vi "ReadInitParameters.vi"(8 "error in (no error)":errorcluster, 11 "INI Filepath":path) -> (0 "error out":errorcluster, 3 "Init Parameters":T1)   [LabVIEW 2020, in "ClashRoyale.lvclass"]
uses:
  ClashRoyale.lvclass
  InitParameters.ctl
  <vilib>/Utility/config.llb/Read Key (String).vi
  <vilib>/Utility/config.llb/NI_LVConfig.lvlib
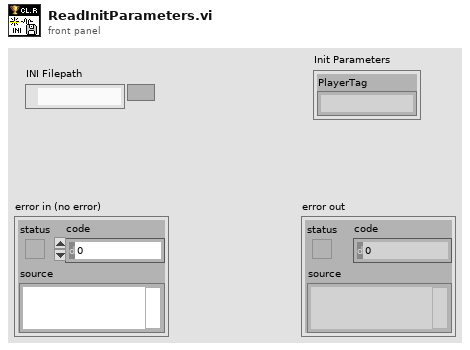
[diagram p1: front panel]
types:
  T1 = typedef "InitParameters.ctl" = cluster{"PlayerTag":string}
  T2 = typedef "NI_LVConfig.lvlib/Config Data RefNum.ctl" = refnum<k1>
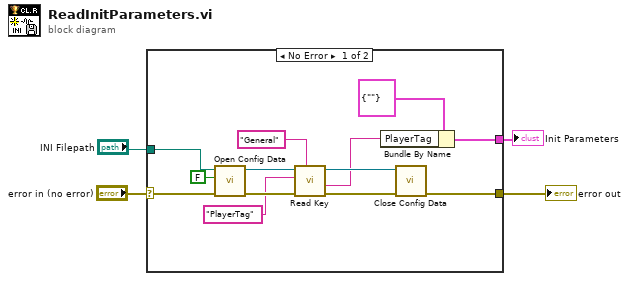
[diagram p0: block diagram]
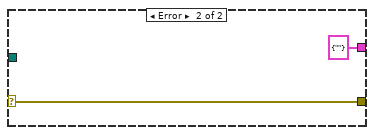
[diagram p2: hidden frame]
diagram:
  n1 = case shown="No Error" "error in (no error)" {
    selector: "error in (no error)" -> [w9 w19]
    tunnel: "INI Filepath" -> [w17 _]
    tunnel: [w8 w19] -> w2
    tunnel: [w5 T1 {"PlayerTag"=""} ("Init Parameters")] -> w1
    frame No Error {
      n2 = call <vilib>:"Open Config Data.vi"("error in (no error)"=w9, "create file if necessary (T)"=FALSE, "configuration file path"=w17) -> ("error out"=w14:errorcluster, "refnum"=w15:T2)  [unwired: 6 in, 1 out]
      n3 = call-poly <vilib>:"Read Key.vi"("section"="General", "error in (no error)"=w14, "key"="PlayerTag", "refnum"=w15) -> ("error out"=w10:errorcluster, "value"=w6:string, "refnum out"=w11:T2)  [unwired: 4 in, 1 out]
      n4 = Bundle By Name(cluster=T1 {"PlayerTag"=""} ("Init Parameters"), "PlayerTag"=w6) -> (w5:T1)
      n5 = call <vilib>:"Close Config Data.vi"("error in (no error)"=w10, "refnum"=w11) -> ("error out"=w8:errorcluster)  [unwired: 8 in, 1 out]
    }
    frame Error {
    }
  }
  "Init Parameters" <- w1
  "error out" <- w2
